vi "Javascript Page Source.vi"() -> ()   [LabVIEW 2020]
uses:
  Webview2 Control/WebView2 Control.xctl
panel:
  out "Document Source 2":string
  in  "stop":bool
  in  "Navigate":bool
  out "WebView2 Control":string(xcontrol)
  in  "URL":string="http://ni.com"
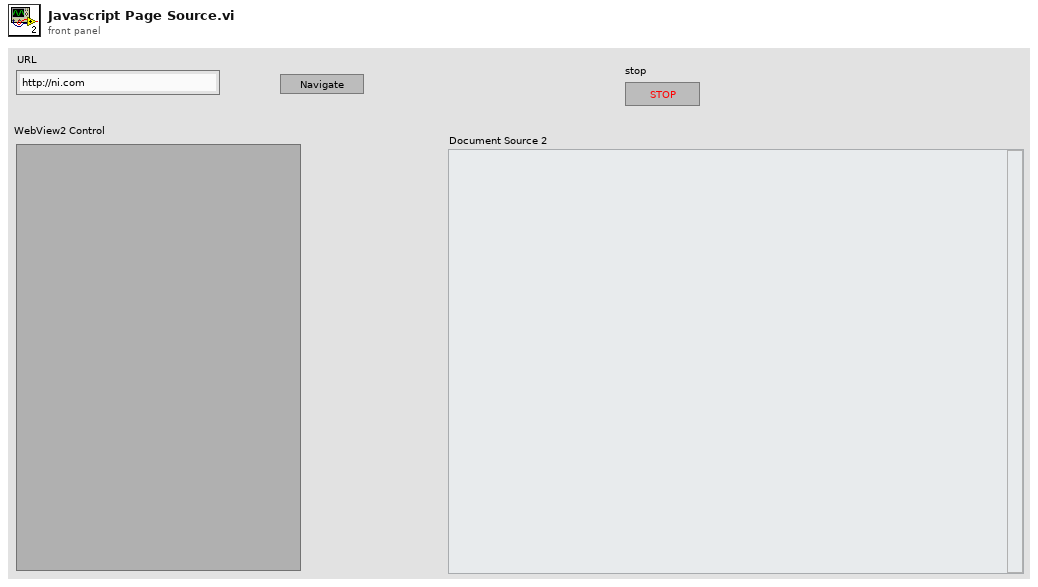
[diagram p1: front panel]
types:
  T1 = typedef "WebView2 Control.xctl/Events.ctl" = cluster{"Navigation Complete Event":refnum<user-event>, "Source Changed Event":refnum<user-event>, "Document Title Changed Event":refnum<user-event>, "Status Bar Text Changed":refnum<user-event>, "Web Message Received":refnum<user-event>, "Window Close Requested":refnum<user-event>, "DOM Loaded":refnum<user-event>}
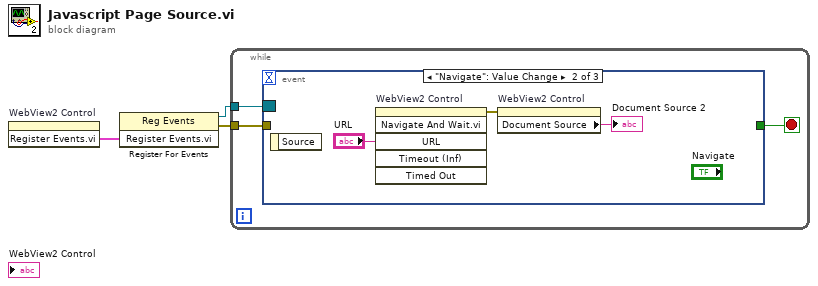
[diagram p0: block diagram]
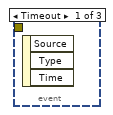
[diagram p2: hidden frame]
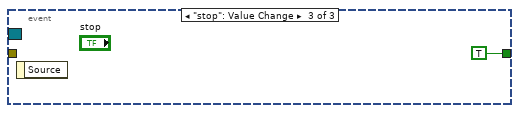
[diagram p3: hidden frame]
diagram:
  n1 = invoke on="WebView2 Control" class="WebView2 Control (strict)" method="Register Events.vi"() -> ("Register Events.vi"=w3:T1)  [unwired: 3 in, 2 out]
  n2 = register-events(w3) -> (reference out=w2:refnum<event-registration>, error out=w1:errorcluster)  [unwired: 2 in]
  n3 = while {
    tunnel: w2 -> [w6]
    tunnel: w1 -> [w5]
    stop <- w4 stop-if-true
    n4 = event shown="[1] \"Navigate\": Value Change" {
      selector: w6 -> [_ _ _]
      dyn-events: _ -> [_ _ _]
      timeout: _ -> [_ _ _]
      tunnel: w5 -> [_ _ _]
      tunnel: [_ _ TRUE] -> w4
      event Timeout {
        n5 = event-data() -> ()  [unwired: 1 in, 3 out]
      }
      event "Navigate": Value Change {
        n6 = event-data() -> ()  [unwired: 1 in, 1 out]
        n7 = invoke on="WebView2 Control" class="WebView2 Control (strict)" method="Navigate And Wait.vi"("URL"="URL") -> (error out=w7:errorcluster)  [unwired: 5 in, 5 out]
        n8 = property on="WebView2 Control" class="WebView2 Control (strict)"(error in=w7) -> ("Document Source"=→"Document Source 2":string)  [unwired: 1 in, 2 out]
      }
      event "stop": Value Change {
        n9 = event-data() -> ()  [unwired: 1 in, 1 out]
      }
    }
  }
